vi "Main.vi"() -> ()   [LabVIEW 2020]
uses:
  <vilib>/MakerHub/LINX/Public/Peripherals/Digital/Digital Write 1 Chan.vi
  85dc64f8-0c24-45cc-aa0c-93b1526429bf.vi
  c2bf3191-8e22-471d-bb4b-7cfb67bb49d1.vi
  <vilib>/MakerHub/LINX/Public/Peripherals/Digital/Digital Write N Chans.vi
  <vilib>/Array/Sort 2D Array - Pop Stack.vi
  <vilib>/Array/Sort 2D Array - Push Stack.vi
  85dc64f8-0c24-45cc-aa0c-93b1526429bf.vi/269d4b3b-47f5-49e3-8884-44851e4dd9d5.vi
  85dc64f8-0c24-45cc-aa0c-93b1526429bf.vi/6d99389c-673d-4efb-bf33-19b32bcf4cf8.vi
  c2bf3191-8e22-471d-bb4b-7cfb67bb49d1.vi/269d4b3b-47f5-49e3-8884-44851e4dd9d5.vi
  c2bf3191-8e22-471d-bb4b-7cfb67bb49d1.vi/6d99389c-673d-4efb-bf33-19b32bcf4cf8.vi
  <vilib>/MakerHub/LINX/Private/Local IO/LinxDigitalWrite.vi
  <vilib>/MakerHub/LINX/Public/Utilities/Check Channel.vi
  <vilib>/MakerHub/LINX/Public/Utilities/Open Serial.vi
  <vilib>/MakerHub/LINX/Private/Utilties/Generate Error.vi
  <vilib>/Utility/file.llb/Read Delimited Spreadsheet (DBL).vi
  <vilib>/MakerHub/LINX/LMH-LINX.lvlib
panel:
  in  "Open existing data Incidence":bool
  in  "Open existing data IV":bool
  in  "Incedence Path":path
  in  "IV Path":path
  out "Fill Factor":dbl
  out "Rsh":dbl
  out "Rs":dbl
  out "Voc":dbl
  out "Isc":dbl
  out "n":dbl
  in  "Serial Port":refnum<visa-resource-name>="N/A"
  out "Angle of Incidence vs Relative Intensity":T1(graph)
  in  "Num Points":i32=50
  out "IV curve":cluster{"PD Voltage":dbl[], "PD Current":dbl[]}(graph)
  in  "Number of Points":dbl=10.0
  in  "Bright/Dark":bool
  in  "Angle of Incedence Test":bool
  in  "IV Trace":bool
  # "NEED TO ADD FILE SAVING FOR ANGLE AND SUPPORT FOR LOADING\nOLD FILES"
  # "Load Existing Data"
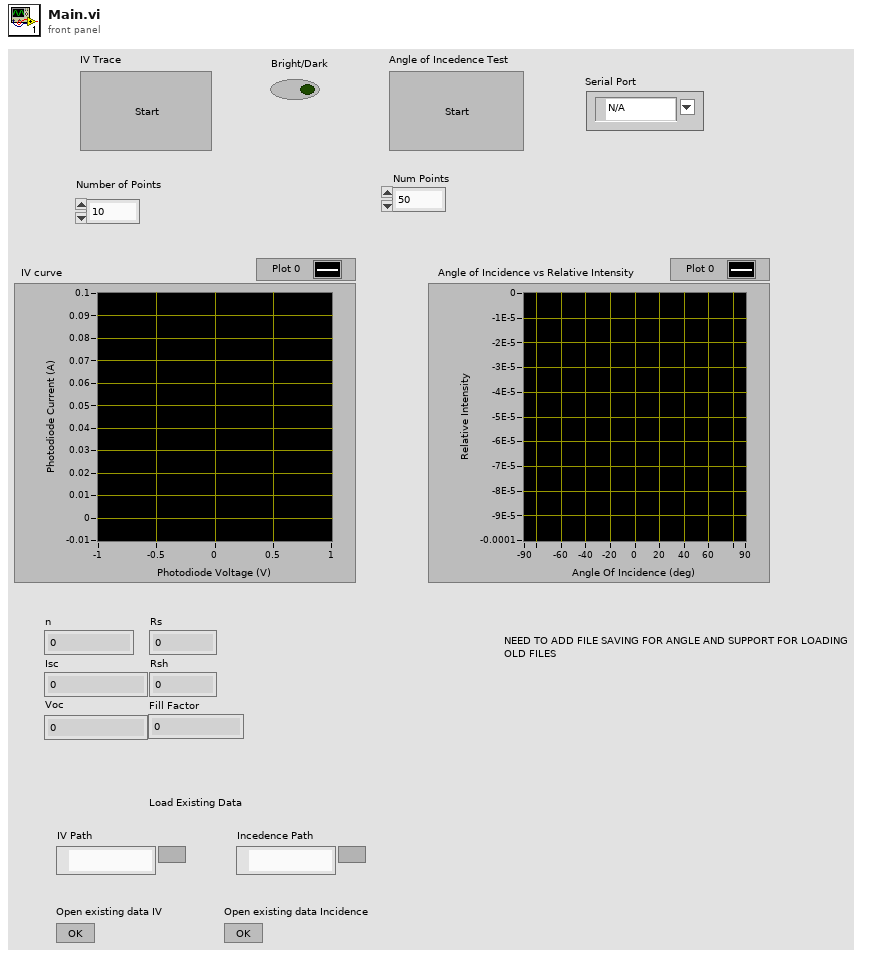
[diagram p1: front panel]
types:
  T1 = cluster{"Incidence angle (deg)":dbl[], "PD current (A)":dbl[]}
  T2 = enum16{"open", "replace", "create", "open or create", "replace or create", "replace or create with confirmation"}
  T3 = typedef "LMH-LINX.lvlib/LINX Ref.ctl" = cluster{"IO":T4, "Interface":T5, "LINX Device Config":T6}
  T4 = typedef "LMH-LINX.lvlib/Platform.ctl" = enum16{"Remote", "Local"}
  T5 = typedef "LMH-LINX.lvlib/Interface.ctl" = enum16{"Serial", "TCP"}
  T6 = typedef "LMH-LINX.lvlib/Device.lvlib/LINX Device Config.ctl" = cluster{"Interface":T5, "COM Port":refnum<visa-resource-name>, "TCP Configuration":T7, "Device Family":u8, "Device ID":u8, "Device Name":string, "TCP Ref":refnum<k5>, "Channels":T8}
  T7 = typedef "LMH-LINX.lvlib/Device.lvlib/TCP Config.ctl" = cluster{"IP Address":string, "Port":u16}
  T8 = typedef "LMH-LINX.lvlib/Channels.ctl" = cluster{"DI":u8[], "DO":u8[], "AI":u8[], "AO":u8[], "PWM":u8[], "QE":u8[], "UART":u8[], "I2C 2":u8[], "SPI":u8[], "CAN":u8[], "Servo":u8[], "AI Ref (V)":dbl, "AI Resolution (Bits)":u8, "AO Ref (V)":dbl, "AO Resolution (Bits)":u8}
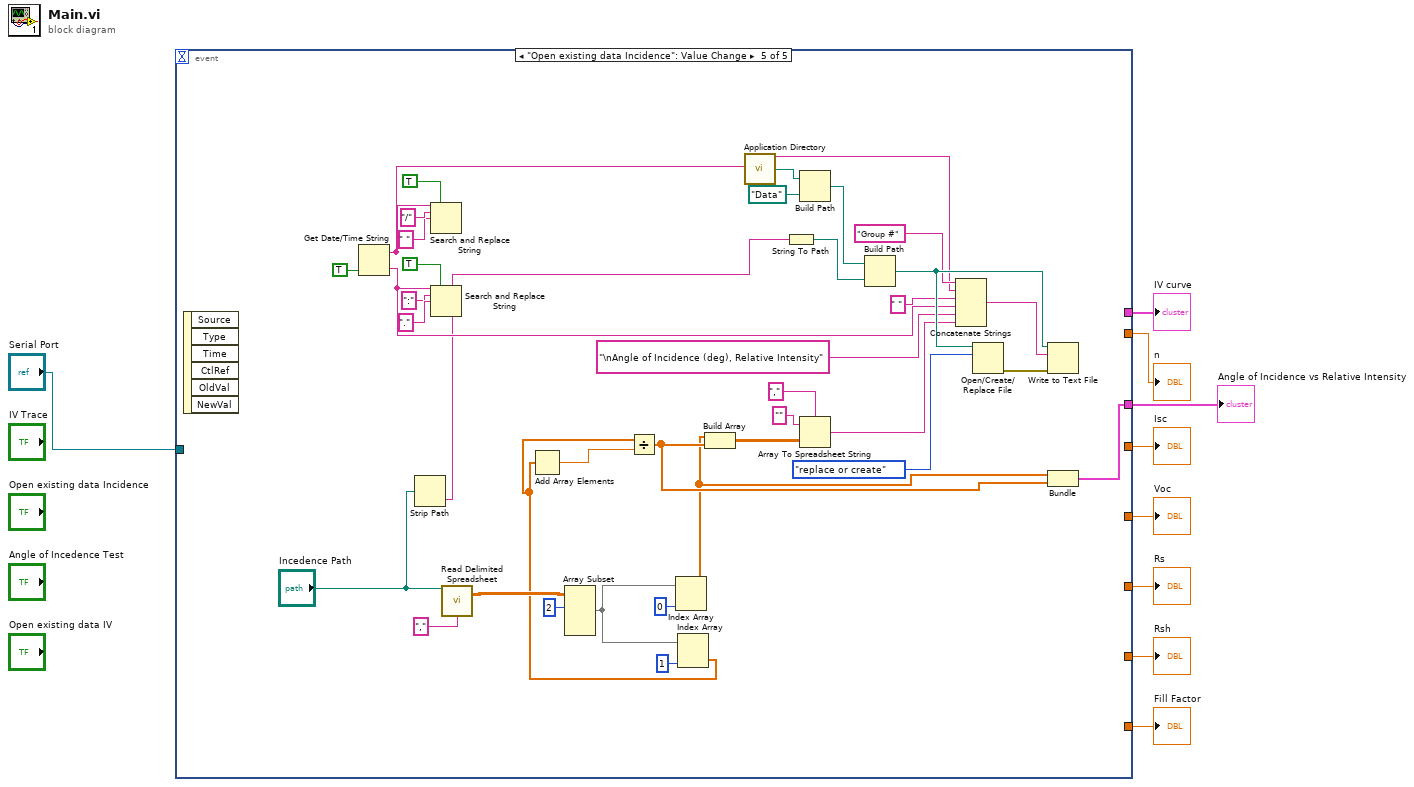
[diagram p0: block diagram]
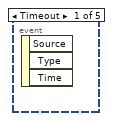
[diagram p2: hidden frame]
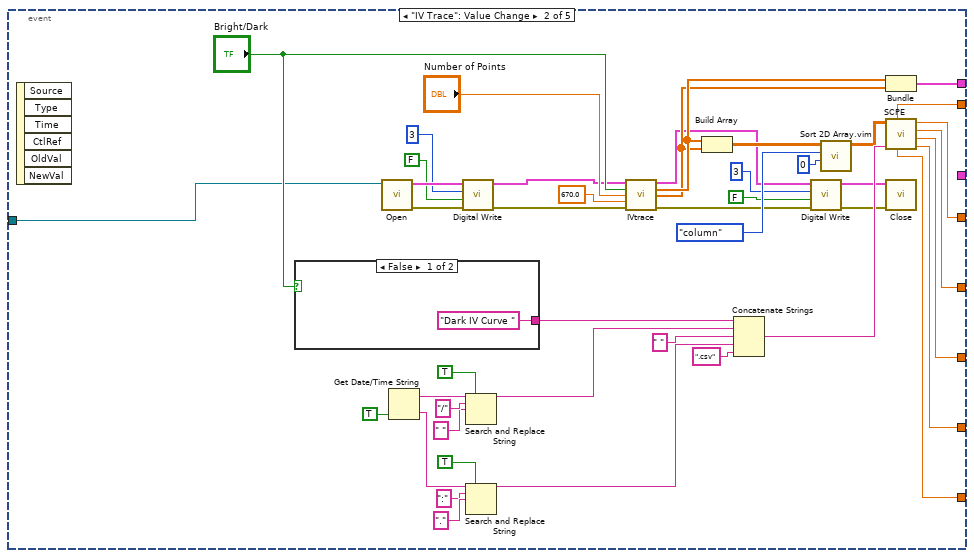
[diagram p3: hidden frame]
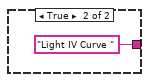
[diagram p4: hidden frame]
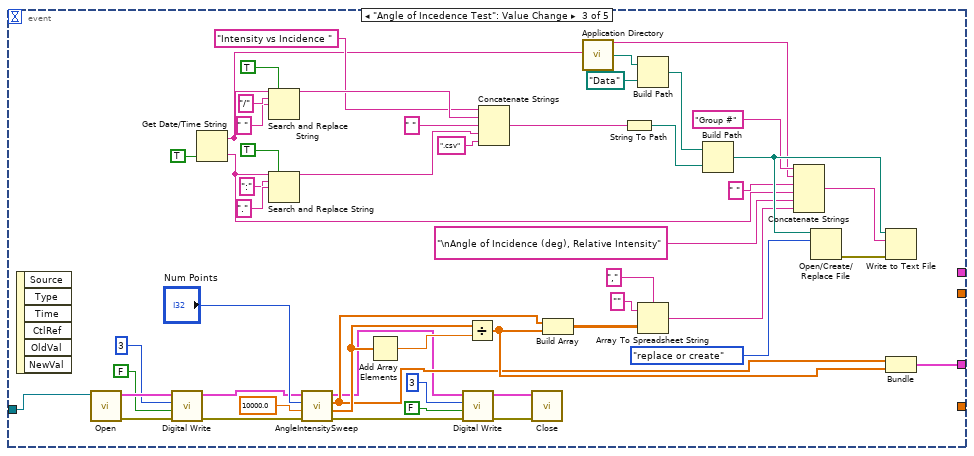
[diagram p5: hidden frame]
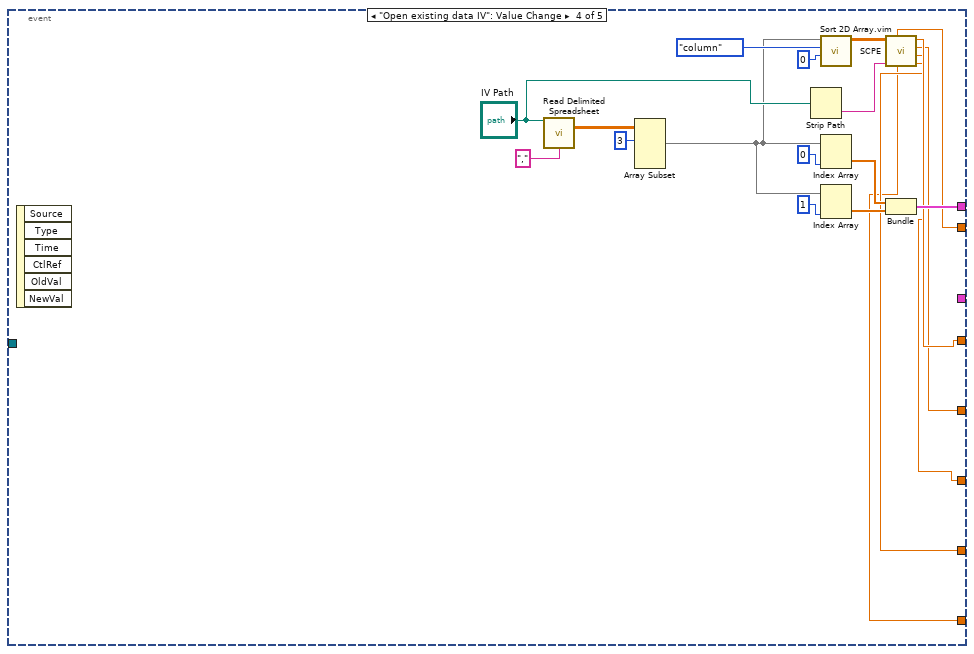
[diagram p6: hidden frame]
diagram:
  n1 = event shown="[4] \"Open existing data Incidence\": Value Change" {
    selector: _ -> [_ _ _ _ _]
    dyn-events: _ -> [_ _ _ _ _]
    timeout: _ -> [_ _ _ _ _]
    tunnel: [_ w49 _ w111 _] -> w9
    tunnel: [_ w48 _ w110 _] -> w8
    tunnel: [_ w47 _ w108 _] -> w7
    tunnel: [_ w46 _ w107 _] -> w6
    tunnel: [_ w45 _ w106 _] -> w5
    tunnel: [_ w44 _ w109 _] -> w4
    tunnel: [_ w43 _ w115 _] -> w3
    tunnel: [_ _ w104 _ w128] -> w2
    tunnel: "Serial Port" -> [_ w10 w56 _ _]
    event Timeout {
      n2 = event-data() -> ()  [unwired: 1 in, 3 out]
    }
    event "IV Trace": Value Change {
      n3 = event-data() -> ()  [unwired: 1 in, 6 out]
      n4 = case shown="False" "Bright/Dark" {
        tunnel: ["Dark IV Curve " "Light IV Curve "] -> w28
        frame False {
        }
        frame True {
        }
      }
      n5 = call-poly <vilib>:"Open.vi"("Serial Port"=w10) -> ("Error Out"=w21:errorcluster, "LINX Resource"=w22:T3)  [unwired: 8 in, 1 out]
      n6 = Get Date/Time String(want seconds? (F)=TRUE) -> (date string=w41:string, time string=w33:string)  [unwired: 2 in]
      n7 = call-poly <vilib>:"Digital Write.vi"("Error In"=w21, "Output Value"=FALSE, "DO Channel"=u8 3, "LINX Resource"=w22) -> ("Error Out"=w18:errorcluster, "LINX Resource"=w17:T3)  [unwired: 6 in]
      n8 = Search and Replace String(replace all?=TRUE ("replace all? (F)"), input string=w41, search string="/" ("substring (\"\")"), replace string=" " ("replace string (\"\")")) -> (result string=w37:string)  [unwired: 4 in, 3 out]
      n9 = Search and Replace String(replace all?=TRUE ("replace all? (F)"), input string=w33, search string=":" ("substring (\"\")"), replace string="." ("replace string (\"\")")) -> (result string=w30:string)  [unwired: 4 in, 3 out]
      n10 = call "IVtrace.vi"("LINX Resource"=w17, "LED On"="Bright/Dark", "Voltage Steps"="Number of Points", "Rf"=670.0, "error in (no error)"=w18) -> ("LINX Resource 2"=w13:T3, "PD Voltage"=w51:dbl[], "PD Current"=w50:dbl[], "Error Out"=w14:errorcluster)  [unwired: 7 in]
      n11 = Build Array(w51, w50) -> (w24:dbl[][])
      n12 = Concatenate Strings(w28, w37, " " ("string"), w30, ".csv" ("string")) -> (w27:string)
      n13 = call-poly <vilib>:"Digital Write.vi"("Error In"=w14, "Output Value"=FALSE, "DO Channel"=u8 3, "LINX Resource"=w13) -> ("Error Out"=w15:errorcluster, "LINX Resource"=w16:T3)  [unwired: 6 in]
      n14 = call "Sort 2D Array.vim"("index"=0, "dimension to index (column)"=enum16{"column", "row"}."column", "2D array"=w24) -> ("sorted 2D array"=w23:dbl[][])  [unwired: 7 in, 1 out]
      n15 = Bundle("PD Voltage"=w51, "PD Current"=w50) -> (w43:cluster{"PD Voltage":dbl[], "PD Current":dbl[]})  [unwired: 1 in]
      n16 = call "SCPE.vi"("FileName"=w27, "IV array"=w23) -> ("Rsh"=w46:dbl, "Rs"=w47:dbl, "Voc"=w44:dbl, "Isc"=w49:dbl, "Fill Factor"=w45:dbl, "n"=w48:dbl)  [unwired: 3 in]
      n17 = call <vilib>:"Close.vi"("Error In"=w15, "LINX Resource"=w16) -> ()  [unwired: 9 in, 1 out]
    }
    event "Angle of Incedence Test": Value Change {
      n18 = event-data() -> ()  [unwired: 1 in, 6 out]
      n19 = call-poly <vilib>:"Open.vi"("Serial Port"=w56) -> ("Error Out"=w68:errorcluster, "LINX Resource"=w67:T3)  [unwired: 8 in, 1 out]
      n20 = call-poly <vilib>:"Digital Write.vi"("Error In"=w68, "Output Value"=FALSE, "DO Channel"=u8 3, "LINX Resource"=w67) -> ("Error Out"=w63:errorcluster, "LINX Resource"=w64:T3)  [unwired: 6 in]
      n21 = Get Date/Time String(want seconds? (F)=TRUE) -> (date string=w76:string, time string=w74:string)  [unwired: 2 in]
      n22 = Search and Replace String(replace all?=TRUE ("replace all? (F)"), input string=w76, search string="/" ("substring (\"\")"), replace string=" " ("replace string (\"\")")) -> (result string=w99:string)  [unwired: 4 in, 3 out]
      n23 = Search and Replace String(replace all?=TRUE ("replace all? (F)"), input string=w74, search string=":" ("substring (\"\")"), replace string="." ("replace string (\"\")")) -> (result string=w93:string)  [unwired: 4 in, 3 out]
      n24 = call "AngleIntensitySweep.vi"("error in (no error)"=w63, "Rf"=10000.0, "Num Points"="Num Points", "LINX Resource"=w64) -> ("Error Out"=w57:errorcluster, "PD Current (A)"=w83:dbl[], "Angle"=w80:dbl[], "LINX Resource 2"=w58:T3)  [unwired: 4 in]
      n25 = Add Array Elements(numeric array=w83) -> (sum=w82:dbl)
      n26 = call-poly <vilib>:"Digital Write.vi"("Error In"=w57, "Output Value"=FALSE, "DO Channel"=u8 3, "LINX Resource"=w58) -> ("Error Out"=w59:errorcluster, "LINX Resource"=w60:T3)  [unwired: 6 in]
      n27 = Divide(x=w83, y=w82) -> (x/y=w81:dbl[])
      n28 = Concatenate Strings("Intensity vs Incidence ", w99, " " ("string"), w93, ".csv" ("string")) -> (w85:string)
      n29 = call <vilib>:"Close.vi"("Error In"=w59, "LINX Resource"=w60) -> ()  [unwired: 9 in, 1 out]
      n30 = Build Array(w80, w81) -> (w79:dbl[][])
      n31 = call <vilib>:"Application Directory.vi"() -> ("Application Directory"=w89:path)
      n32 = String To Path(string=w85) -> (path=w87:path)
      n33 = Build Path(base path=w89, name or relative path=path "Data") -> (appended path=w88:path)
      n34 = Array To Spreadsheet String(delimiter (Tab)=",", array=w79, 3:"" ("format string")) -> (spreadsheet string=w72:string)
      n35 = Build Path(base path=w88, name or relative path=w87) -> (appended path=w84:path)
      n36 = Concatenate Strings("Group #" ("string"), w76, " " ("string"), w74, "\nAngle of Incidence (deg), Relative Intensity" ("string"), w72) -> (w71:string)
      n37 = Open/Create/Replace File(file path (use dialog)=w84, operation (0:open)=T2."replace or create") -> (error out=w70:errorcluster)  [unwired: 4 in, 2 out]
      n38 = Write to Text File(file (use dialog)=w84, text=w71, error in=w70) -> ()  [unwired: 1 in, 3 out]
      n39 = Bundle("Angle"=w80, w81) -> (w104:cluster{"Angle":dbl[], dbl[]})  [unwired: 1 in]
    }
    event "Open existing data IV": Value Change {
      n40 = event-data() -> ()  [unwired: 1 in, 6 out]
      n41 = call-poly <vilib>:"Read Delimited Spreadsheet.vi"("file path (dialog if empty)"="IV Path", "delimiter (\\t)"="," ("delimiter (\\t)")) -> ("all rows"=w121:dbl[][])  [unwired: 8 in, 5 out]
      n42 = Array Subset(array=w121, index (row)=3 ("index")) -> (w112:dbl[][])  [unwired: 3 in]
      n43 = Strip Path(path="IV Path") -> (name=w122:string)  [unwired: 1 out]
      n44 = call "Sort 2D Array.vim"("index"=0, "dimension to index (column)"=enum16{"column", "row"}."column", "2D array"=w112) -> ("sorted 2D array"=w120:dbl[][])  [unwired: 7 in, 1 out]
      n45 = Index Array(array=w112, index (col)=0 ("disabled index (col)")) -> (element=w117:dbl[])  [unwired: 1 in]
      n46 = Index Array(array=w112, index (col)=1 ("disabled index (col)")) -> (element=w116:dbl[])  [unwired: 1 in]
      n47 = call "SCPE.vi"("FileName"=w122, "IV array"=w120) -> ("Rsh"=w107:dbl, "Rs"=w108:dbl, "Voc"=w109:dbl, "Isc"=w111:dbl, "Fill Factor"=w106:dbl, "n"=w110:dbl)  [unwired: 3 in]
      n48 = Bundle(w117, w116) -> (w115:cluster{dbl[], dbl[]})  [unwired: 1 in]
    }
    event "Open existing data Incidence": Value Change {
      n49 = event-data() -> ()  [unwired: 1 in, 6 out]
      n50 = Get Date/Time String(want seconds? (F)=TRUE) -> (date string=w144:string, time string=w142:string)  [unwired: 2 in]
      n51 = Strip Path(path="Incedence Path") -> (name=w126:string)  [unwired: 1 out]
      n52 = Search and Replace String(replace all?=TRUE ("replace all? (F)"), input string=w144, search string="/" ("substring (\"\")"), replace string=" " ("replace string (\"\")")) -> ()  [unwired: 4 in, 4 out]
      n53 = Search and Replace String(replace all?=TRUE ("replace all? (F)"), input string=w142, search string=":" ("substring (\"\")"), replace string="." ("replace string (\"\")")) -> ()  [unwired: 4 in, 4 out]
      n54 = call-poly <vilib>:"Read Delimited Spreadsheet.vi"("file path (dialog if empty)"="Incedence Path", "delimiter (\\t)"="," ("delimiter (\\t)")) -> ("all rows"=w134:dbl[][])  [unwired: 8 in, 5 out]
      n55 = Array Subset(array=w134, index (row)=2 ("index")) -> (w133:dbl[][])  [unwired: 3 in]
      n56 = Index Array(array=w133, index (col)=0 ("disabled index (col)")) -> (element=w129:dbl[])  [unwired: 1 in]
      n57 = Index Array(array=w133, index (col)=1 ("disabled index (col)")) -> (element=w130:dbl[])  [unwired: 1 in]
      n58 = Add Array Elements(numeric array=w130) -> (sum=w149:dbl)
      n59 = Divide(x=w130, y=w149) -> (x/y=w148:dbl[])
      n60 = Build Array(w129, w148) -> (w147:dbl[][])
      n61 = call <vilib>:"Application Directory.vi"() -> ("Application Directory"=w154:path)
      n62 = String To Path(string=w126) -> (path=w152:path)
      n63 = Build Path(base path=w154, name or relative path=path "Data") -> (appended path=w153:path)
      n64 = Array To Spreadsheet String(delimiter (Tab)=",", array=w147, 3:"" ("format string")) -> (spreadsheet string=w140:string)
      n65 = Build Path(base path=w153, name or relative path=w152) -> (appended path=w150:path)
      n66 = Concatenate Strings("Group #" ("string"), w144, " " ("string"), w142, "\nAngle of Incidence (deg), Relative Intensity" ("string"), w140) -> (w139:string)
      n67 = Open/Create/Replace File(file path (use dialog)=w150, operation (0:open)=T2."replace or create") -> (error out=w138:errorcluster)  [unwired: 4 in, 2 out]
      n68 = Write to Text File(file (use dialog)=w150, text=w139, error in=w138) -> ()  [unwired: 1 in, 3 out]
      n69 = Bundle(w129, w148) -> (w128:cluster{dbl[], dbl[]})  [unwired: 1 in]
    }
  }
  "Isc" <- w9
  "n" <- w8
  "Rs" <- w7
  "Rsh" <- w6
  "Fill Factor" <- w5
  "Voc" <- w4
  "IV curve" <- w3
  "Angle of Incidence vs Relative Intensity" <- w2
